vi "easing_QuintInOut.vi"(9 "distance":dbl, 10 "interval (10 ms)":dbl, 11 "time":dbl) -> (3 "current position":dbl)   [LabVIEW 2023]
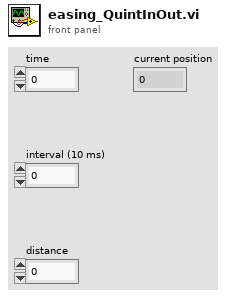
[diagram p1: front panel]
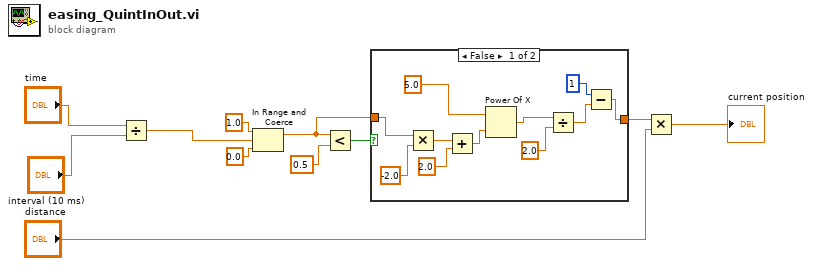
[diagram p0: block diagram]
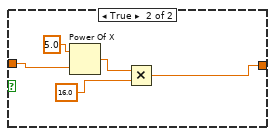
[diagram p2: hidden frame]
diagram:
  n1 = Divide(x="time", y="interval (10 ms)") -> (x/y=w5:dbl)
  n2 = In Range and Coerce(upper limit=1.0, x=w5, lower limit=0.0 ("upper limit")) -> (coerced(x)=w2:dbl)  [unwired: 1 out]
  n3 = Less?(x=w2, y=0.5) -> (x < y?=w4:bool)
  n4 = case shown="False" w4 {
    tunnel: w2 -> [w15 w27]
    tunnel: [w19 w23] -> w1
    frame False {
      n5 = Multiply(x=w15, y=-2.0) -> (x*y=w14:dbl)
      n6 = Add(x=w14, y=2.0) -> (x+y=w13:dbl)
      n7 = Power Of X(1:w13, 2:5.0 ("y")) -> (0:w17:dbl)
      n8 = Divide(x=w17, y=2.0) -> (x/y=w21:dbl)
      n9 = Subtract(x=1, y=w21) -> (x-y=w19:dbl)
    }
    frame True {
      n10 = Power Of X(1:w27, 2:5.0 ("y")) -> (0:w24:dbl)
      n11 = Multiply(x=w24, y=16.0) -> (x*y=w23:dbl)
    }
  }
  n12 = Multiply(x=w1, y="distance") -> (x*y=→"current position":dbl)
